vi "Rate Limiter.vi"(10 "Increment Array":dbl[](array[numeric]), 11 "Input Array":dbl[](array[numeric])) -> (3 "Output Array":dbl[](array[numeric]))   [LabVIEW 2010]
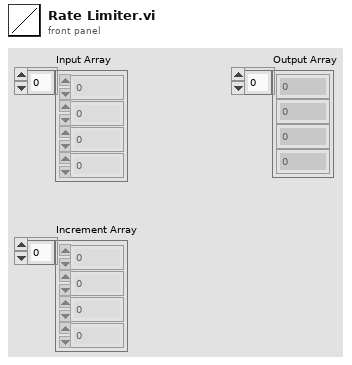
[diagram p1: front panel]
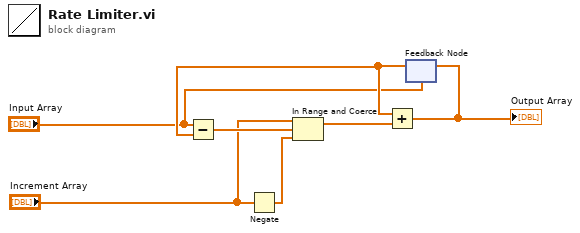
[diagram p0: block diagram]
diagram:
  n1 = Negate(x="Increment Array") -> (-x=w7:dbl[])
  n2 = feedback #1("Input Array") -> (w5:dbl[])
  n3 = Subtract(x="Input Array", y=w5) -> (x-y=w4:dbl[])
  n4 = In Range and Coerce(upper limit="Increment Array", x=w4, lower limit=w7) -> (coerced(x)=w6:dbl[])  [unwired: 1 out]
  n5 = Add(x=w5, y=w6) -> (x+y=w1:dbl[])
  "Output Array" <- w1
  n6 = feedback-in #1(w1) -> ()
